vi "getSelfPath.vi"(0 "reference":refnum<class "BentStyle.lvclass">, 1 "bounds":T2 {"height" format="%.2f"; "width" format="%.2f"; "y" format="%.2f"; "x" format="%.2f"}, 5 "error in (no error)":errorcluster) -> (14 "reference out":refnum<class "BentStyle.lvclass">, 15 "path":T1[](array[typedef]) {"y" format="%.2f"; "x" format="%.2f"}, 19 "error out":errorcluster)   [LabVIEW 2014, in "BentStyle.lvclass"]
doc: "private static ArrayList getSelfPath(Rectangle2D s)"
uses:
  <resource>/Framework/Providers/Open_GDS/UML/BentStyle_class/BentStyle.lvclass
  <resource>/Framework/Providers/Open_GDS/UML/General/Rectangle/Rectangle Rectangle2D.ctl
  <resource>/Framework/Providers/Open_GDS/UML/General/Point/Point Point2D.ctl
  <resource>/Framework/Providers/Open_GDS/UML/BentStyle_class/BentStyle.lvclass/BentStyle.ctl
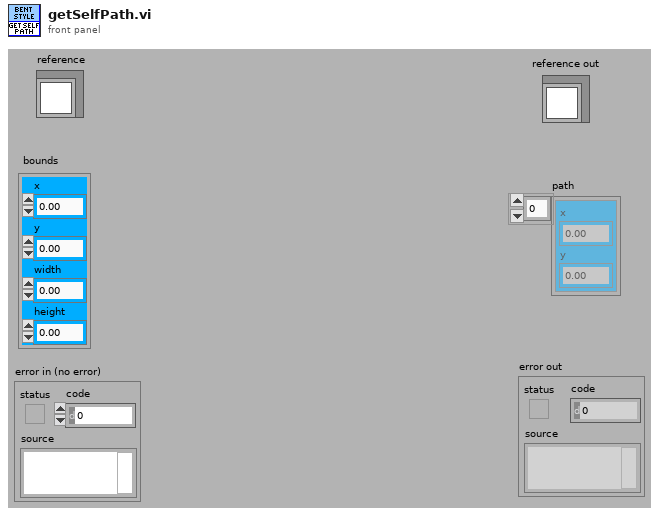
[diagram p1: front panel]
types:
  T1 = typedef "Point Point2D.ctl" = cluster{"x":dbl, "y":dbl}
  T2 = typedef "Rectangle Rectangle2D.ctl" = cluster{"x":dbl, "y":dbl, "width":dbl, "height":dbl}
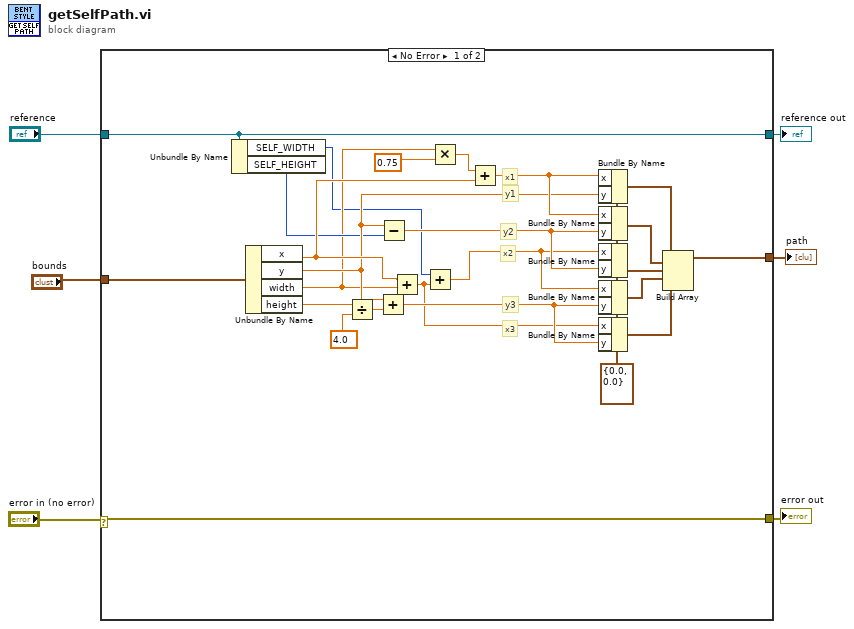
[diagram p0: block diagram]
diagram:
  n1 = case shown="No Error" "error in (no error)" {
    selector: "error in (no error)" -> [w7 w32]
    tunnel: "reference" -> [w8 w33]
    tunnel: [w7 w32] -> w5
    tunnel: [w8 w33] -> w4
    tunnel: "bounds" -> [w31 _]
    tunnel: [w30 _] -> w1
    frame No Error {
      w29 = T1 {"x"=0.0, "y"=0.0} ("point2D")
      # "x3"
      # "y3"
      # "x2"
      # "y2"
      # "y1"
      # "x1"
      n2 = Unbundle By Name(w8) -> ("SELF_WIDTH"=w9:i32, "SELF_HEIGHT"=w14:i32)
      n3 = Unbundle By Name(w31) -> ("x"=w20:dbl, "y"=w15:dbl, "width"=w10:dbl, "height"=w13:dbl)
      n4 = Divide(x=w13, y=4.0) -> (x/y=w16:dbl)
      n5 = Add(x=w15, y=w16) -> (x+y=w12:dbl)
      n6 = Subtract(x=w15, y=w14) -> (x-y=w19:dbl)
      n7 = Add(x=w20, y=w10) -> (x+y=w11:dbl)
      n8 = Add(x=w9, y=w11) -> (x+y=w18:dbl)
      n9 = Multiply(x=w10, y=0.75) -> (x*y=w22:dbl)
      n10 = Add(x=w22, y=w20) -> (x+y=w21:dbl)
      n11 = Bundle By Name(cluster=w29, "x"=w21, "y"=w15) -> (w28:T1)
      n12 = Bundle By Name(cluster=w29, "x"=w21, "y"=w19) -> (w27:T1)
      n13 = Bundle By Name(cluster=w29, "x"=w18, "y"=w19) -> (w26:T1)
      n14 = Bundle By Name(cluster=w29, "x"=w18, "y"=w12) -> (w25:T1)
      n15 = Bundle By Name(cluster=w29, "x"=w11, "y"=w12) -> (w24:T1)
      n16 = Build Array(w28, w27, w26, w25, w24) -> (w30:T1[])
    }
    frame Error {
    }
  }
  "reference out" <- w4
  "error out" <- w5
  "path" <- w1
